vi "Calculate equalization FIR.vi"(0 "channel":T1, 5 "FIR taps":i32=32, 7 "Max FIR gain":dbl=6.0) -> (4 "EQ FIR coeff":cdb[](array[numeric]), 6 "Mag response":cluster{"xi used":dbl[], "yi":dbl[]}[](graph), 8 "Phase response":cluster{"xi used":dbl[], "yi":dbl[]}(graph))   [LabVIEW 2019]
uses:
  <vilib>/Analysis/1siggen.llb/Ramp Pattern by Samples.vi
  <vilib>/Analysis/2dsp.llb/Inverse Complex FFT.vi
  <vilib>/Analysis/4window.llb/Hamming Window (CDB).vi
  <vilib>/Analysis/4window.llb/AllCosWindow (CDB).vi
  <vilib>/Analysis/NI_AALBase.lvlib
  <vilib>/gmath/NI_Gmath.lvlib
  <vilib>/Analysis/NI_AALPro.lvlib
panel:
  out "FIR coeff graph":dbl[][](graph)
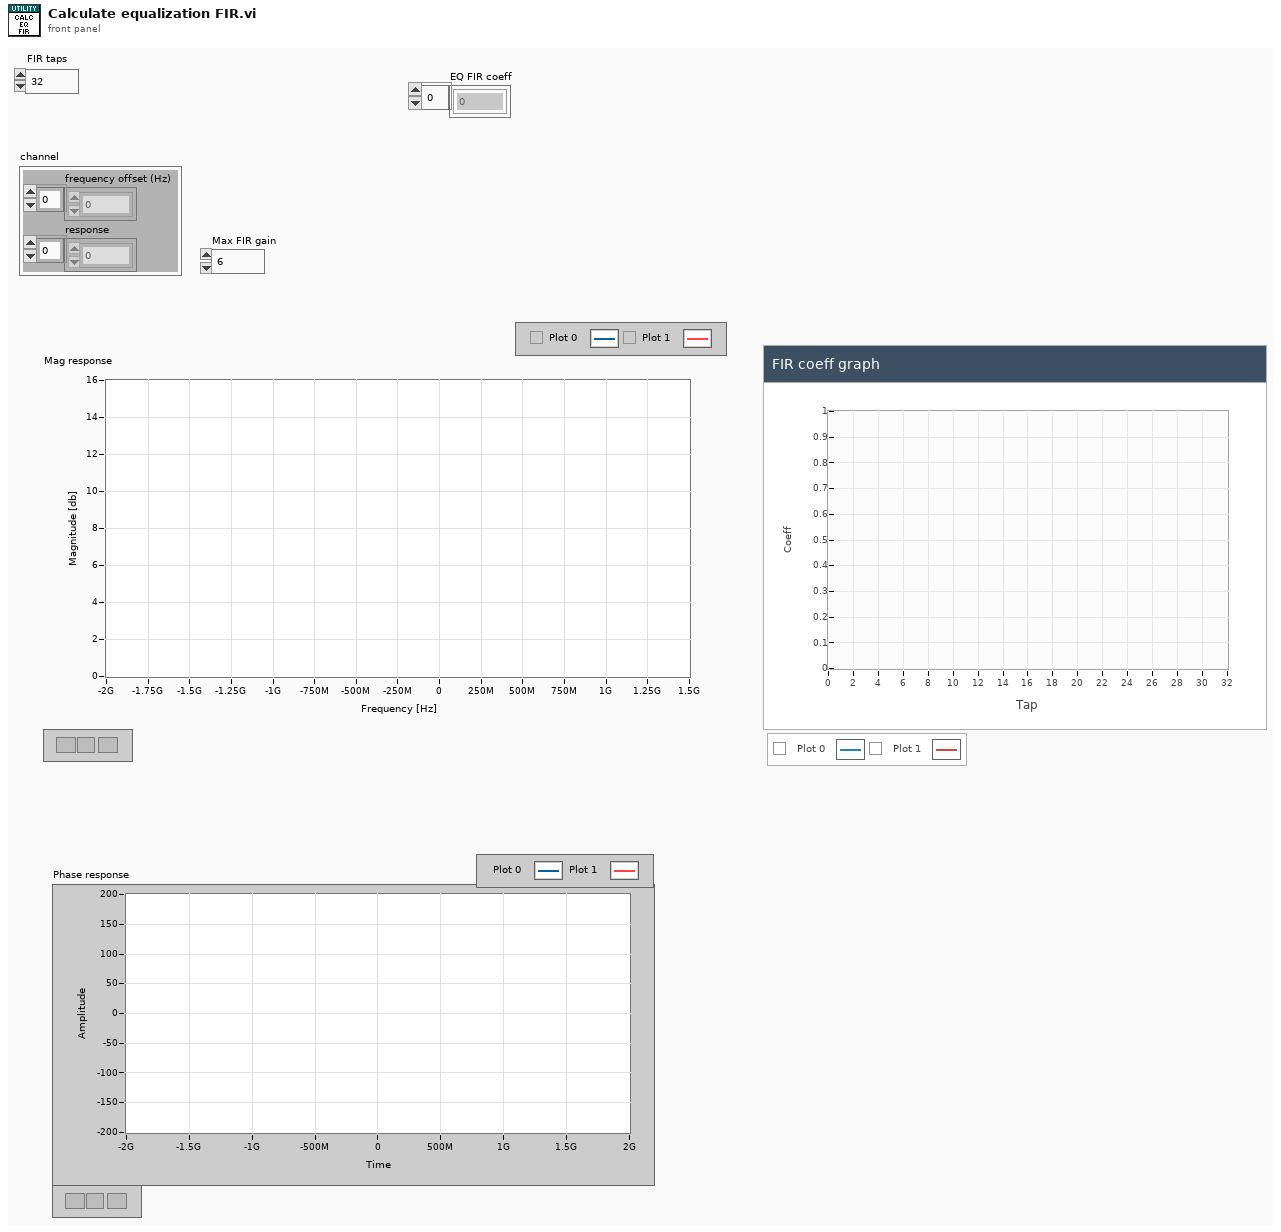
[diagram p1: front panel]
types:
  T1 = cluster{"frequency offset (Hz)":dbl[], "response":cdb[]}
  T2 = typedef "Constants.ctl" = cluster{"data clock rate (Hz)":dbl, "sample rate (Hz)":dbl, "sample rate selector string":string, "default tx bitfile path":path, "default rx bitfile path":path, "default proc bitfile path":path}
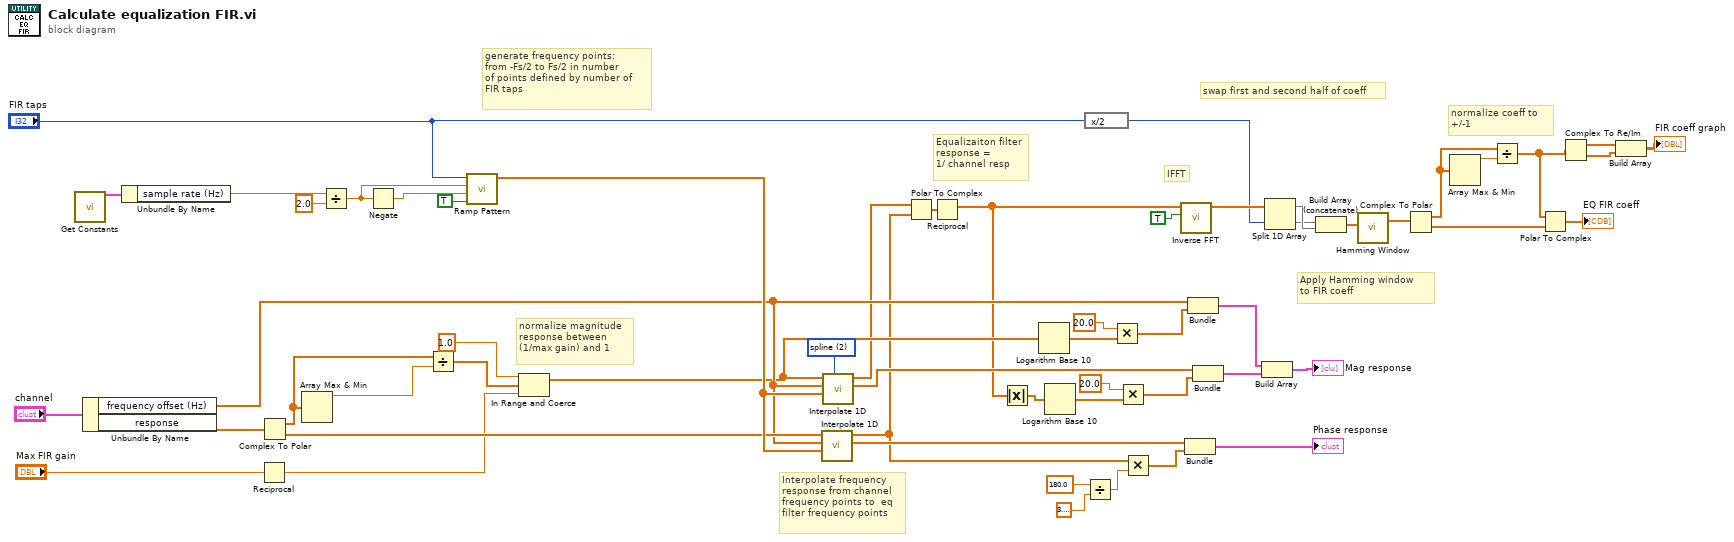
[diagram p0: block diagram]
diagram:
  w51 = 2 items=["nearest", "linear", "spline", "cubic Hermite", "Lagrange"] ("method")
  # "Apply Hamming window\nto FIR coeff"
  # "swap first and second half of coeff"
  # "IFFT"
  # "Equalizaiton filter\nresponse =\n1/ channel resp"
  # "normalize magnitude\nresponse between\n(1/max gain) and 1"
  # "Interpolate frequency\nresponse from channel\nfrequency points to  eq\nfilter frequency points"
  # "generate frequency points:\nfrom -Fs/2 to Fs/2 in number\nof points defined by number of\nFIR taps"
  # "normalize coeff to +/-1"
  n1 = call "Get Constants.vi"() -> ("constants"=w23:T2)  [unwired: 15 in]
  n2 = Unbundle By Name("channel") -> ("frequency offset (Hz)"=w41:dbl[], "response"=w43:cdb[])
  n3 = Unbundle By Name(w23) -> ("sample rate (Hz)"=w22:dbl)
  n4 = Reciprocal(x="Max FIR gain") -> (1/x=w19:dbl)
  n5 = Complex To Polar(r * e^(i*theta)=w43) -> (r=w39:dbl[], theta=w42:dbl[])
  n6 = Array Max & Min(array=w39) -> (max value=w40:dbl)  [unwired: 3 out]
  n7 = Divide(x=w22, y=2.0) -> (x/y=w53:dbl)
  n8 = Negate(x=w53) -> (-x=w54:dbl)
  n9 = Divide(x=w39, y=w40) -> (x/y=w37:dbl[])
  n10 = call-poly <vilib>:"Ramp Pattern.vi"("exclude end?"=TRUE, "start"=w54, "end"=w53, "samples"="FIR taps") -> ("Ramp Pattern"=w50:dbl[])  [unwired: 6 in, 1 out]
  n11 = In Range and Coerce(upper limit=1.0, x=w37, lower limit=w19) -> (coerced(x)=w34:dbl[])  [unwired: 1 out]
  n12 = call <vilib>:"Interpolate 1D.vi"("xi"=w50, "X"=w41, "Y"=w42) -> ("xi used"=w45:dbl[], "yi"=w25:dbl[])  [unwired: 6 in, 1 out]
  n13 = call <vilib>:"Interpolate 1D.vi"("method"=w51, "xi"=w50, "X"=w41, "Y"=w34) -> ("xi used"=w49:dbl[], "yi"=w30:dbl[])  [unwired: 5 in, 1 out]
  n14 = Polar To Complex(1:w25, 2:w30) -> (0:w21:cdb[])
  n15 = Reciprocal(x=w21) -> (1/x=w11:cdb[])
  n16 = Absolute Value(x=w11) -> (abs(x)=w10:dbl[])
  n17 = Logarithm Base 10(1:w34) -> (0:w36:dbl[])
  n18 = Logarithm Base 10(1:w10) -> (0:w31:dbl[])
  n19 = expression code="x/2"("FIR taps") -> (w16:i32)
  n20 = Divide(x=180.0, y=3.141592653589793) -> (x/y=w26:dbl)
  n21 = Multiply(x=20.0, y=w36) -> (x*y=w33:dbl[])
  n22 = Multiply(x=20.0, y=w31) -> (x*y=w29:dbl[])
  n23 = Multiply(x=w25, y=w26) -> (x*y=w24:dbl[])
  n24 = call-poly <vilib>:"Inverse FFT.vi"("shift?"=TRUE, "FFT {X}"=w11) -> ("X"=w17:cdb[])  [unwired: 8 in, 1 out]
  n25 = Bundle("xi used"=w45, w24) -> (→"Phase response":cluster{"xi used":dbl[], dbl[]})  [unwired: 1 in]
  n26 = Bundle("frequency offset (Hz)"=w41, w33) -> (w47:cluster{"frequency offset (Hz)":dbl[], dbl[]})  [unwired: 1 in]
  n27 = Bundle("xi used"=w49, w29) -> (w48:cluster{"xi used":dbl[], dbl[]})  [unwired: 1 in]
  n28 = Build Array(w47, w48) -> (→"Mag response":cluster{"xi used":dbl[], dbl[]}[])
  n29 = Split 1D Array(array=w17, index=w16) -> (first subarray=w15:cdb[], second subarray=w14:cdb[])
  n30 = Build Array (concatenate)(w14, w15) -> (w13:cdb[])
  n31 = call-poly <vilib>:"Hamming Window.vi"("X"=w13) -> ("Windowed X"=w8:cdb[])  [unwired: 1 out]
  n32 = Complex To Polar(r * e^(i*theta)=w8) -> (r=w9:dbl[], theta=w7:dbl[])
  n33 = Array Max & Min(array=w9) -> (max value=w5:dbl)  [unwired: 3 out]
  n34 = Divide(x=w9, y=w5) -> (x/y=w4:dbl[])
  n35 = Polar To Complex(1:w7, 2:w4) -> (0:→"EQ FIR coeff":cdb[])
  n36 = Complex To Re/Im(x + iy=w4) -> (x=w3:dbl[], y=w1:dbl[])
  n37 = Build Array(w3, w1) -> (→"FIR coeff graph":dbl[][])
